vi "Channel Setting.vi"(8 "error in (no error)":errorcluster, 11 "Node Ptr":T1 format="%.0x") -> (0 "error out":errorcluster)   [LabVIEW 2017, in "Serial Communcation Devices Custom Device.lvlib"]
uses:
  Serial Communcation Devices Custom Device.lvlib
  <vilib>/NI Veristand/Custom Device API/Custom Device Item Ref.ctl
  <vilib>/NI Veristand/Custom Device API/Get Item Property (String).vi
  <vilib>/NI Veristand/Custom Device API/Set Item Property (Variant).vi
  <vilib>/NI Veristand/Custom Device API/Set Item Property (U16).vi
  <vilib>/NI Veristand/Custom Device API/Set Item Property (U32).vi
  <vilib>/NI Veristand/Custom Device API/Get Item Property (U16).vi
  <vilib>/NI Veristand/Custom Device API/Custom Device API.lvlib
panel:
  in  "parity":u16(ring) items=["None", "Odd", "Even", "Mark", "Space"]
  in  "stop bits":u16(ring)=10 items=["1.0"=10, "1.5"=15, "2.0"=20]
  in  "flow control":u16(ring) items=["None"=0, "XON/XOFF"=1, "RTS/CTS"=2, "DTR/DSR"=4]
  in  "baud rate 2":u32=9600
  in  "data bits":u16=8 min=5 max=8 step=1
  in  "VISA resource name":refnum<visa-resource-name>
  out "Parity":dbl
  out "VISA Resource Name":string
  out "Flow Control":dbl
  out "Stop bits":dbl
  out "Data bits":dbl
  out "Baud rate":dbl
  out "Timeout":dbl
  out "Enable Termination Char":bool
  in  "Header":cluster{"Section Name":string}={"Section Name"="Custom Device Item Settings"}
  in  "Description":string
  in  "Name":string
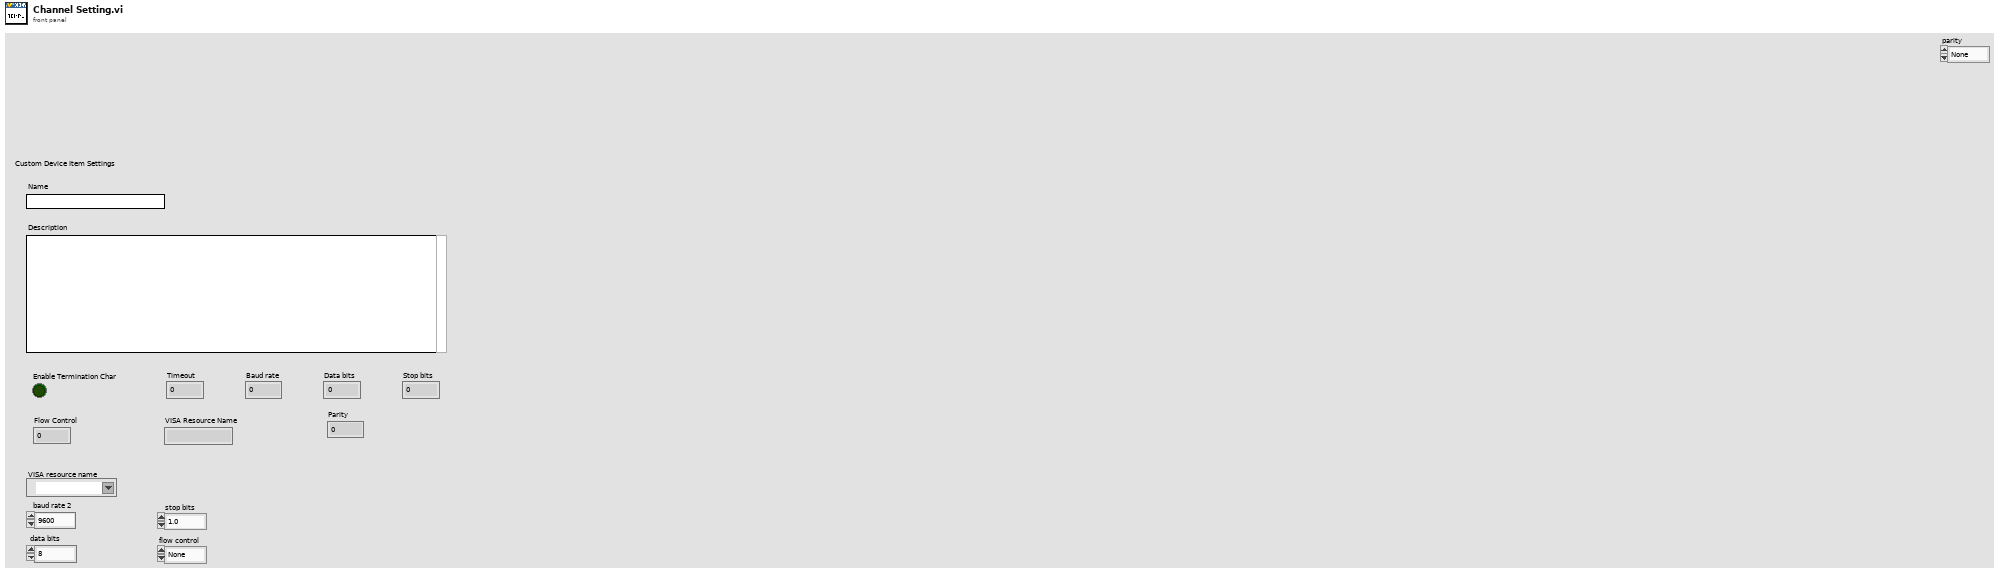
[diagram p1: front panel]
types:
  T1 = typedef "Custom Device API.lvlib/Custom Device Item Ref.ctl" = u64
  T2 = typedef "Custom Device API.lvlib/Custom Device Item Info.ctl" = cluster{"Name":string, "Is Channel":bool, "GUID":string, "Is Waveform":bool}
  T3 = typedef "Custom Device API.lvlib/Custom Device Commands.ctl" = enum16{"Default", "Item renamed", "Shutdown", "Dynamic button pressed"}
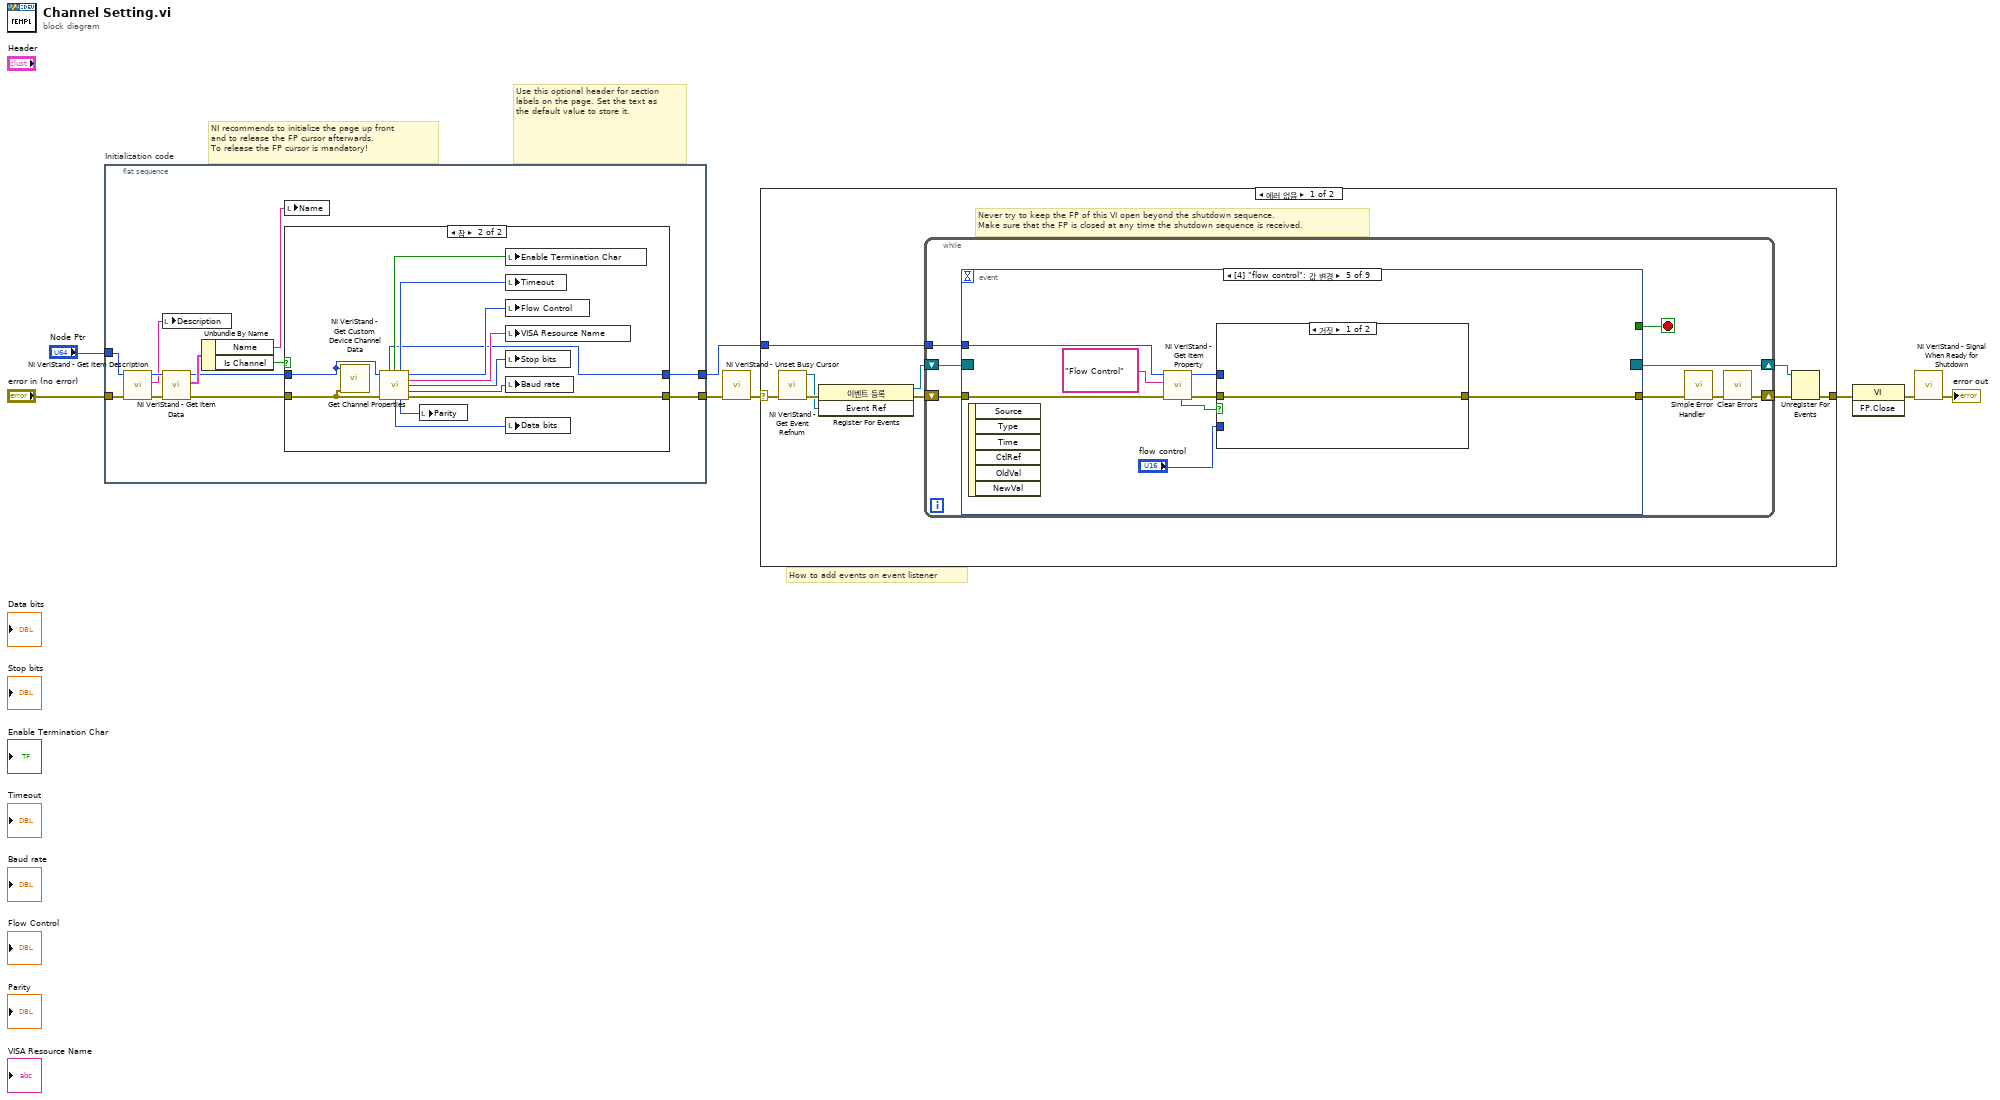
[diagram p0: block diagram]
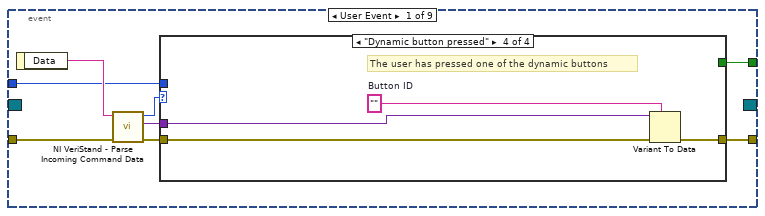
[diagram p2: hidden frame]
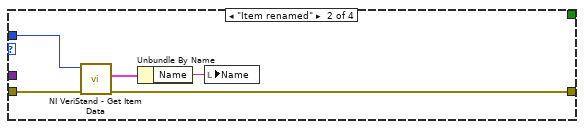
[diagram p4: hidden frame]
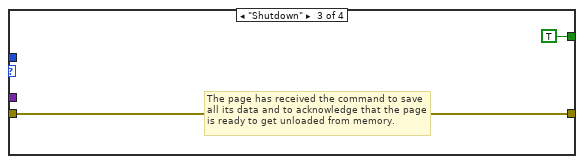
[diagram p5: hidden frame]
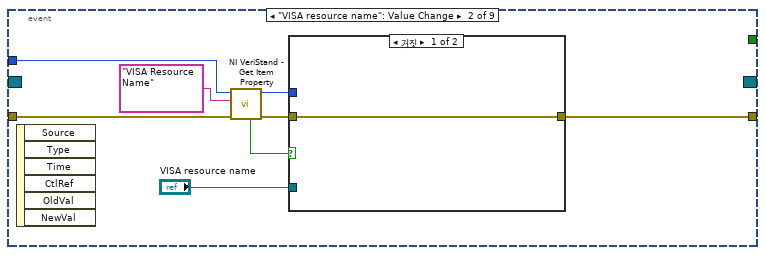
[diagram p6: hidden frame]
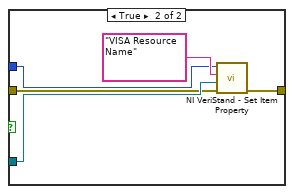
[diagram p7: hidden frame]
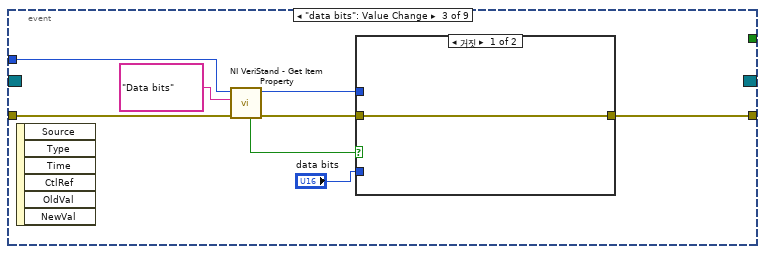
[diagram p8: hidden frame]
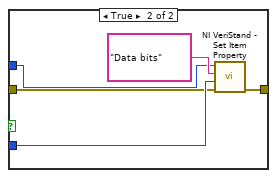
[diagram p9: hidden frame]
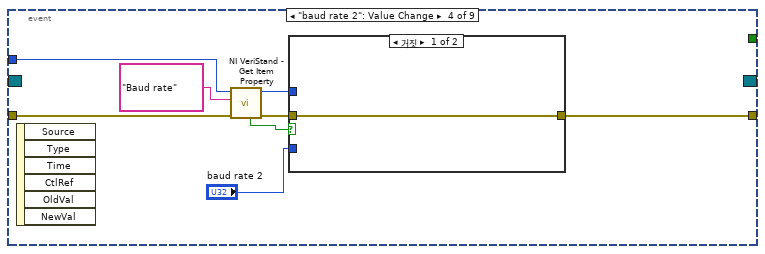
[diagram p10: hidden frame]
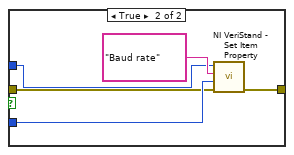
[diagram p11: hidden frame]
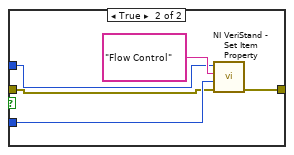
[diagram p12: hidden frame]
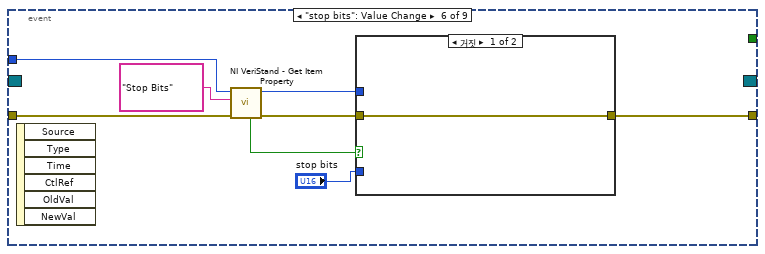
[diagram p13: hidden frame]
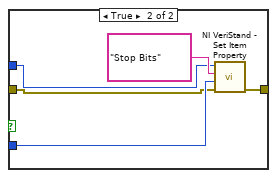
[diagram p14: hidden frame]
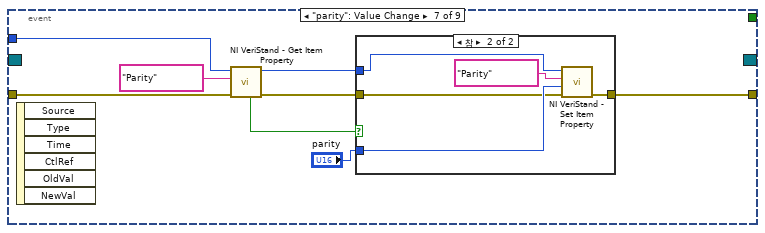
[diagram p15: hidden frame]
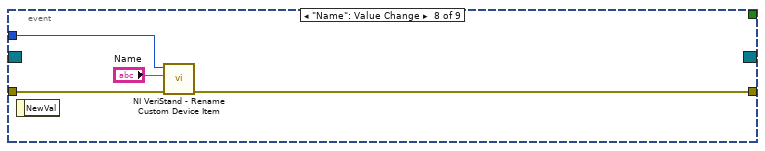
[diagram p17: hidden frame]
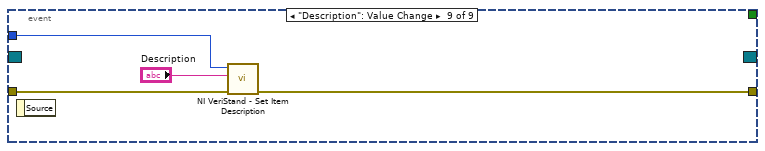
[diagram p18: hidden frame]
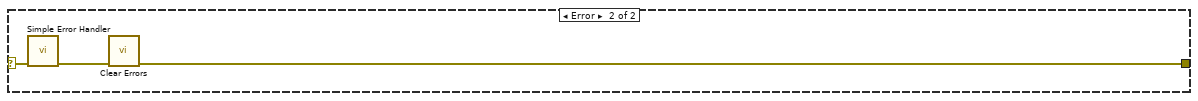
[diagram p19: hidden frame]
diagram:
  # "How to add events on event listener"
  # "Use this optional header for section labels on the page. Set the text as the default value to store it."
  # "NI recommends to initialize the page up front\nand to release the FP cursor afterwards.\nTo release the FP cursor is mandatory!"
  n1 = flat-sequence "Initialization code" {
    tunnel: "error in (no error)" -> [w19]
    tunnel: "Node Ptr" -> [w18]
    tunnel: [w11] -> w4
    tunnel: [w12] -> w1
    frame #0 {
      n2 = call <vilib>:"NI VeriStand - Get Item Description.vi"("error in (no error)"=w19, "Item Ref in"=w18) -> ("error out"=w16:errorcluster, "Description"=w17:string, "Item Ref out"=w20:T1)  [unwired: 7 out]
      n3 = local write "Description"(w17) -> ()
      n4 = call <vilib>:"NI VeriStand - Get Item Data.vi"("error in (no error)"=w16, "Item Ref in"=w20) -> ("error out"=w10:errorcluster, "Item Info"=w15:T2, "Item Ref out"=w13:T1)  [unwired: 7 out]
      n5 = Unbundle By Name(w15) -> ("Name"=w14:string, "Is Channel"=w9:bool)
      n6 = local write "Name"(w14) -> ()
      n7 = case shown="참" w9 {
        tunnel: w13 -> [w22 w33]
        tunnel: [w22 w23] -> w12
        tunnel: [w21 w24] -> w11
        tunnel: w10 -> [w21 w34]
        frame False {
        }
        frame True {
          n8 = call <vilib>:"NI VeriStand - Get Custom Device Channel Data.vi"("error in (no error)"=w34, "Channel Ref in"=w33) -> ()  [unwired: 4 in, 6 out]
          n9 = call "Get Channel Properties.vi"("Item Ref In"=w33, "에러 입력(에러 없음)"=w34) -> ("Item Ref out"=w23:T1, "Enable Termination Char"=w32:bool, "Timeout"=w31:u16, "Flow Control"=w25:u16, "VISA\nResource\nName"=w30:string, "Stop Bits"=w26:u16, "Baud rate"=w29:u16, "Data bits"=w28:u16, "Parity"=w27:u16, "에러 출력"=w24:errorcluster)  [unwired: 4 in]
          n10 = local write "Parity"(w27) -> ()
          n11 = local write "Enable Termination Char"(w32) -> ()
          n12 = local write "Timeout"(w31) -> ()
          n13 = local write "Flow Control"(w25) -> ()
          n14 = local write "VISA Resource Name"(w30) -> ()
          n15 = local write "Stop bits"(w26) -> ()
          n16 = local write "Baud rate"(w29) -> ()
          n17 = local write "Data bits"(w28) -> ()
        }
      }
    }
  }
  n18 = call <vilib>:"NI VeriStand - Unset Busy Cursor.vi"("error in (no error)"=w4) -> ("error out"=w3:errorcluster)  [unwired: 10 out]
  n19 = case shown="에러 없음" w3 {
    selector: w3 -> [w35 w166]
    tunnel: [w40 w164] -> w8
    tunnel: w1 -> [w36 _]
    frame No Error {
      # "Never try to keep the FP of this VI open beyond the shutdown sequence.\nMake sure that the FP is closed at any time the shutdown sequence is received."
      n20 = call <vilib>:"NI VeriStand - Get Event Refnum.vi"("error in (no error)"=w35) -> ("error out"=w43:errorcluster, "Event Ref"=w39:refnum<user-event>)  [unwired: 9 out]
      n21 = register-events(error in=w43, w39) -> (reference out=w37:refnum<event-registration>, error out=w38:errorcluster)  [unwired: 1 in]
      n22 = while {
        tunnel: w36 -> [w47]
        shift-right: [w44] -> w41
        shift-left: w38 -> [w50]
        shift-right: [w51] -> w42
        shift-left: w37 -> [w49]
        stop <- w48 stop-if-true
        n23 = event shown="[4] \"flow control\": 값 변경" {
          selector: w49 -> [_ _ _ _ _ _ _ _ _]
          dyn-events: [_ _ _ _ _ _ _ _ _] -> w51
          timeout: _ -> [_ _ _ _ _ _ _ _ _]
          tunnel: w50 -> [w59 w72 w88 w102 w115 w130 w148 w159 w162]
          tunnel: [w55 _ _ _ _ _ _ _ _] -> w48
          tunnel: [w54 w74 w87 w100 w116 w128 w145 w158 w161] -> w46
          tunnel: w47 -> [w53 w75 w89 w103 w114 w129 w144 w157 w163]
          event User Event {
            n24 = event-data() -> ("Data"=w58:string)  [unwired: 1 out]
            n25 = call <vilib>:"NI VeriStand - Parse Incoming Command Data.vi"("error in (no error)"=w59, "Incoming data"=w58) -> ("error out"=w57:errorcluster, "Outgoing data"=w52:variant, "Action"=w56:T3)  [unwired: 7 out]
            n26 = case shown="\"Dynamic button pressed\"" w56 {
              tunnel: w57 -> [w60 w65 w66 w71]
              tunnel: [_ _ TRUE _] -> w55
              tunnel: [w60 w62 w66 w68] -> w54
              tunnel: w53 -> [_ w64 _ _]
              tunnel: w52 -> [_ _ _ w70]
              frame "Default", Default {
              }
              frame "Item renamed" {
                n27 = call <vilib>:"NI VeriStand - Get Item Data.vi"("error in (no error)"=w65, "Item Ref in"=w64) -> ("error out"=w62:errorcluster, "Item Info"=w63:T2)  [unwired: 8 out]
                n28 = Unbundle By Name(w63) -> ("Name"=w61:string)
                n29 = local write "Name"(w61) -> ()
              }
              frame "Shutdown" {
                # "The page has received the command to save all its data and to acknowledge that the page is ready to get unloaded from memory."
              }
              frame "Dynamic button pressed" {
                w69 = ""  # Button ID
                # "The user has pressed one of the dynamic buttons"
                n30 = Variant To Data(error in=w71, type=w69, Variant=w70) -> (error out=w68:errorcluster)  [unwired: 1 out]
              }
            }
          }
          event "VISA resource name": Value Change {
            n31 = event-data() -> ()  [unwired: 7 out]
            n32 = call-poly <vilib>:"NI VeriStand - Get Item Property.vi"("error in (no error)"=w72, "Property Name"="VISA Resource Name", "Item Ref in"=w75) -> ("error out"=w79:errorcluster, "Item Ref out"=w78:T1, "Found?"=w76:bool)  [unwired: 5 in, 1 out]
            n33 = case shown="거짓" w76 {
              tunnel: "VISA resource name" -> [_ w85]
              tunnel: w79 -> [w80 w81]
              tunnel: w78 -> [_ w83]
              tunnel: [w80 w82] -> w74
              frame False {
              }
              frame True {
                n34 = call-poly <vilib>:"NI VeriStand - Set Item Property.vi"("error in (no error)"=w81, "Value"=w85, "Property Name"="VISA Resource Name", "Item Ref in"=w83) -> ("error out"=w82:errorcluster)  [unwired: 5 in, 2 out]
              }
            }
          }
          event "data bits": Value Change {
            n35 = event-data() -> ()  [unwired: 7 out]
            n36 = call-poly <vilib>:"NI VeriStand - Get Item Property.vi"("error in (no error)"=w88, "Property Name"="Data bits", "Item Ref in"=w89) -> ("error out"=w93:errorcluster, "Item Ref out"=w92:T1, "Found?"=w90:bool)  [unwired: 5 in, 1 out]
            n37 = case shown="거짓" w90 {
              tunnel: "data bits" -> [_ w99]
              tunnel: w93 -> [w94 w95]
              tunnel: w92 -> [_ w97]
              tunnel: [w94 w96] -> w87
              frame False {
              }
              frame True {
                n38 = call-poly <vilib>:"NI VeriStand - Set Item Property.vi"("error in (no error)"=w95, "Value"=w99, "Property Name"="Data bits", "Item Ref in"=w97) -> ("error out"=w96:errorcluster)  [unwired: 5 in, 2 out]
              }
            }
          }
          event "baud rate 2": Value Change {
            n39 = event-data() -> ()  [unwired: 7 out]
            n40 = call-poly <vilib>:"NI VeriStand - Get Item Property.vi"("error in (no error)"=w102, "Property Name"="Baud rate", "Item Ref in"=w103) -> ("error out"=w107:errorcluster, "Item Ref out"=w106:T1, "Found?"=w104:bool)  [unwired: 5 in, 1 out]
            n41 = case shown="거짓" w104 {
              tunnel: "baud rate 2" -> [_ w113]
              tunnel: w107 -> [w108 w109]
              tunnel: w106 -> [_ w111]
              tunnel: [w108 w110] -> w100
              frame False {
              }
              frame True {
                n42 = call-poly <vilib>:"NI VeriStand - Set Item Property.vi"("error in (no error)"=w109, "Value"=w113, "Property Name"="Baud rate", "Item Ref in"=w111) -> ("error out"=w110:errorcluster)  [unwired: 5 in, 2 out]
              }
            }
          }
          event "flow control": Value Change {
            n43 = event-data() -> ()  [unwired: 7 out]
            n44 = call-poly <vilib>:"NI VeriStand - Get Item Property.vi"("error in (no error)"=w115, "Property Name"="Flow Control", "Item Ref in"=w114) -> ("error out"=w121:errorcluster, "Item Ref out"=w120:T1, "Found?"=w118:bool)  [unwired: 5 in, 1 out]
            n45 = case shown="거짓" w118 {
              tunnel: "flow control" -> [_ w127]
              tunnel: w121 -> [w122 w125]
              tunnel: w120 -> [_ w124]
              tunnel: [w122 w123] -> w116
              frame False {
              }
              frame True {
                n46 = call-poly <vilib>:"NI VeriStand - Set Item Property.vi"("error in (no error)"=w125, "Value"=w127, "Property Name"="Flow Control", "Item Ref in"=w124) -> ("error out"=w123:errorcluster)  [unwired: 5 in, 2 out]
              }
            }
          }
          event "stop bits": Value Change {
            n47 = event-data() -> ()  [unwired: 7 out]
            n48 = call-poly <vilib>:"NI VeriStand - Get Item Property.vi"("error in (no error)"=w130, "Property Name"="Stop Bits", "Item Ref in"=w129) -> ("error out"=w135:errorcluster, "Item Ref out"=w134:T1, "Found?"=w132:bool)  [unwired: 5 in, 1 out]
            n49 = case shown="거짓" w132 {
              tunnel: "stop bits" -> [_ w141]
              tunnel: w135 -> [w136 w139]
              tunnel: w134 -> [_ w138]
              tunnel: [w136 w137] -> w128
              frame False {
              }
              frame True {
                n50 = call-poly <vilib>:"NI VeriStand - Set Item Property.vi"("error in (no error)"=w139, "Value"=w141, "Property Name"="Stop Bits", "Item Ref in"=w138) -> ("error out"=w137:errorcluster)  [unwired: 5 in, 2 out]
              }
            }
          }
          event "parity": Value Change {
            n51 = event-data() -> ()  [unwired: 7 out]
            n52 = call-poly <vilib>:"NI VeriStand - Get Item Property.vi"("error in (no error)"=w148, "Property Name"="Parity", "Item Ref in"=w144) -> ("error out"=w147:errorcluster, "Item Ref out"=w146:T1, "Found?"=w142:bool)  [unwired: 5 in, 1 out]
            n53 = case shown="참" w142 {
              tunnel: "parity" -> [_ w155]
              tunnel: w147 -> [w150 w151]
              tunnel: w146 -> [_ w153]
              tunnel: [w150 w152] -> w145
              frame False {
              }
              frame True {
                n54 = call-poly <vilib>:"NI VeriStand - Set Item Property.vi"("error in (no error)"=w151, "Value"=w155, "Property Name"="Parity", "Item Ref in"=w153) -> ("error out"=w152:errorcluster)  [unwired: 5 in, 2 out]
              }
            }
          }
          event "Name": Value Change {
            n55 = event-data() -> ()  [unwired: 2 out]
            n56 = call <vilib>:"NI VeriStand - Rename Custom Device Item.vi"("error in (no error)"=w159, "New Name"="Name", "Item Ref in"=w157) -> ("error out"=w158:errorcluster)  [unwired: 1 in, 7 out]
          }
          event "Description": Value Change {
            n57 = event-data() -> ()  [unwired: 2 out]
            n58 = call <vilib>:"NI VeriStand - Set Item Description.vi"("error in (no error)"=w162, "Description"="Description", "Item Ref in"=w163) -> ("error out"=w161:errorcluster)  [unwired: 8 out]
          }
        }
        n59 = call <vilib>:"Simple Error Handler.vi"("error in (no error)"=w46) -> ("error out"=w45:errorcluster)  [unwired: 1 in, 7 out]
        n60 = call <vilib>:"Clear Errors.vi"("error in (no error)"=w45) -> ("error out"=w44:errorcluster)  [unwired: 1 in, 5 out]
      }
      n61 = Unregister For Events(event registration refnum=w42, error in=w41) -> (error out=w40:errorcluster)
    }
    frame Error {
      n62 = call <vilib>:"Simple Error Handler.vi"("error in (no error)"=w166) -> ("error out"=w165:errorcluster)  [unwired: 1 in, 7 out]
      n63 = call <vilib>:"Clear Errors.vi"("error in (no error)"=w165) -> ("error out"=w164:errorcluster)  [unwired: 1 in, 5 out]
    }
  }
  n64 = invoke class="VI" method="FP.Close"(error in=w8) -> (error out=w7:errorcluster)  [unwired: 2 in, 2 out]
  n65 = call <vilib>:"NI VeriStand - Signal When Ready for Shutdown.vi"("error in (no error)"=w7) -> ("error out"=→"error out":errorcluster)  [unwired: 10 out]
